vi "Make Window Always on Top.vi"(4 "error in (no error)":errorcluster, 5 "activate? (F)":bool, 6 "window name (\"\")":string, 7 "window refnum (NaWR)":T1) -> (0 "error out":errorcluster)   [LabVIEW 2026]
doc: "This function will make the window named in the 'window name' input, or identified by the 'window refnum' the topmost window, so it will always be on top of other windows. If 'not a window refnum' is passed in, then the function will use the window name to get a window window refnum. If the window cannot be found, an error will be returned."
uses:
  Actor.lvclass/Actor.ctl
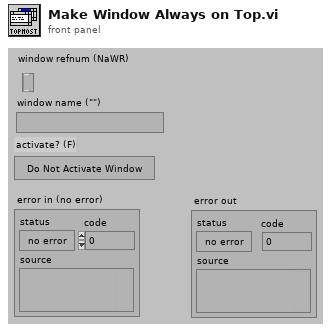
[diagram p1: front panel]
types:
  T1 = typedef "Win32 Util.lvlib/Window Refnum" = refnum<k1>
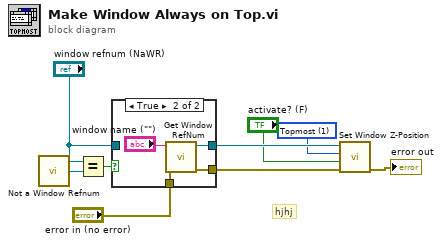
[diagram p0: block diagram]
diagram:
  w2 = i16 1 items=["Not Topmost", "Topmost", "Top", "Bottom"]
  # "hjhj"
  n1 = call "Not a Window Refnum"() -> ("Not a Window Refnum"=w7:T1)
  n2 = Equal?(x="window refnum (NaWR)", y=w7) -> (x = y?=w8:bool)
  n3 = case shown="True" w8 {
    tunnel: "error in (no error)" -> [w10 w15]
    tunnel: [w11 w14] -> w5
    tunnel: "window refnum (NaWR)" -> [w11 _]
    tunnel: [w10 w13] -> w4
    frame False {
    }
    frame True {
      n4 = call "Get Window RefNum.vi"("error in (no error)"=w15, "window name (\"\")"="window name (\"\")") -> ("error out"=w13:errorcluster, "window refnum (NaWR)"=w14:T1)  [unwired: 6 in]
    }
  }
  n5 = call "Set Window Z-Position.vi"("error in (no error)"=w4, "activate? (T)"="activate? (F)", "z-order position"=w2, "window refnum"=w5) -> ("error out"=→"error out":errorcluster)  [unwired: 2 in, 1 out]
